vi "Write IncDec Visible.vi"(5 "IncDec Visible":bool, 9 "Digital in":refnum<class "Digital.lvclass">) -> (3 "Digital out":refnum<class "Digital.lvclass">)   [LabVIEW 2014, in "Digital.lvclass"]
uses:
  Digital.lvclass
  Digital.lvclass/Digital.ctl
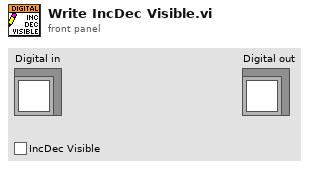
[diagram p1: front panel]
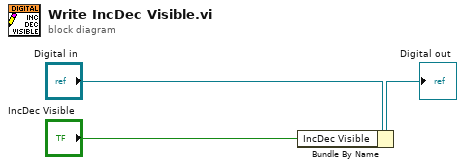
[diagram p0: block diagram]
diagram:
  n1 = Bundle By Name(cluster="Digital in", "IncDec Visible"="IncDec Visible") -> (→"Digital out":refnum<class "Digital.lvclass">)
